vi "Utility Read From Register.vi"(7 "Unit Address (1)":u8=1, 8 "error in (no error)":errorcluster, 9 "Num Of Reg (1)":u16=1 min=1 step=1, 10 "Register Address (0)":u16, 11 "VISA resource name":refnum<visa-resource-name>) -> (0 "error out":errorcluster, 2 "Data":i16[](array[numeric]), 3 "VISA resource name out":refnum<visa-resource-name>)   [LabVIEW 2014, in "Eurotherm 35xx Series.lvlib"]
doc: "This VI reads value from specified registers of specified unit."
uses:
  <instrlib>/Eurotherm 35xx Series/Eurotherm 35xx Series.lvlib
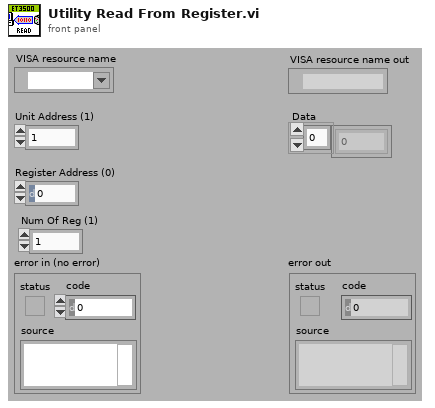
[diagram p1: front panel]
types:
  T1 = enum16{"By The Number of Bytes", "Copy Of the Sent Message"}
  T2 = cluster{"Read Buffer[0]":u8, "Read Buffer[1]":u8}
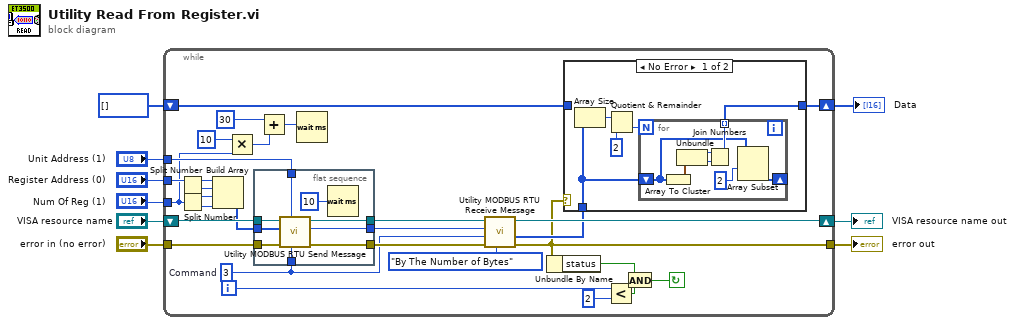
[diagram p0: block diagram]
diagram:
  n1 = while {
    tunnel: "Unit Address (1)" -> [w19]
    shift-right: [w35] -> w8
    shift-left: "VISA resource name" -> [w36]
    tunnel: "Register Address (0)" -> [w25]
    tunnel: "Num Of Reg (1)" -> [w10]
    shift-right: [w23] -> w6
    shift-left: u16[] [] -> [w22]
    tunnel: [w16] -> w2
    tunnel: "error in (no error)" -> [w15]
    i -> [w31]
    stop <- w33 continue-if-true
    w32 = u8 3  # Command
    n2 = Split Number(x=w25) -> (hi(x)=w27:u8, lo(x)=w26:u8)
    n3 = Split Number(x=w10) -> (hi(x)=w21:u8, lo(x)=w20:u8)
    n4 = Build Array(w27, w26, w21, w20) -> (w28:u8[])
    n5 = Multiply(x=u32 10, y=w10) -> (x*y=w13:u32)
    n6 = flat-sequence {
      tunnel: [w47] -> w38
      tunnel: [w46] -> w37
      tunnel: w36 -> [w45]
      tunnel: w32 -> [w44]
      tunnel: w28 -> [w43]
      tunnel: w19 -> [w42]
      tunnel: [w41] -> w17
      tunnel: w15 -> [w40]
      frame #0 {
        n7 = call <instrlib>:"Utility MODBUS RTU Send Message.vi"("Command (0)"=w44, "Unit Address (1)"=w42, "error in (no error)"=w40, "Message (empty array)"=w43, "VISA resource name"=w45) -> ("error out"=w47:errorcluster, "Length Of Sent MSG"=w41:u8, "VISA resource name out"=w46:refnum<visa-resource-name>)  [unwired: 4 in]
        n8 = Wait (ms)(milliseconds to wait=u32 10) -> ()  [unwired: 1 out]
      }
    }
    n9 = Add(x=u32 30 ("milliseconds to wait"), y=w13) -> (x+y=w12:u32)
    n10 = Wait (ms)(milliseconds to wait=w12) -> ()  [unwired: 1 out]
    n11 = call <instrlib>:"Utility MODBUS RTU Receive Message.vi"("Receive Message Type (0: By The Number Of Bytes)"=T1."By The Number of Bytes" ("Receive Message Type"), "error in (no error)"=w38, "Sent Command (0)"=w32, "Length Of Sent MSG (0)"=w17, "VISA resource name"=w37) -> ("error out"=w16:errorcluster, "Read Buffer"=w24:u8[], "VISA resource name out"=w35:refnum<visa-resource-name>)  [unwired: 4 in]
    n12 = Unbundle By Name(w16) -> ("status"=w34:bool)
    n13 = case shown="No Error" w16 {
      tunnel: w24 -> [w52 _]
      tunnel: [w51 w60] -> w23
      tunnel: w22 -> [_ w60]
      frame No Error {
        n14 = Array Size(array=w52) -> (size(s)=w50:i32)
        n15 = Quotient & Remainder(x=w50, y=2) -> (floor(x/y)=w48:i32)  [unwired: 1 out]
        n16 = for {
          N: w48 -> [_]
          shift-right: [w54] -> _
          shift-left: w52 -> [w55]
          tunnel: [w56] -> w51 mode=indexing
          n17 = Array To Cluster(array=w55) -> (cluster=w59:T2)
          n18 = Unbundle(w59) -> ("Read Buffer[0]"=w57:u8, "Read Buffer[1]"=w58:u8)
          n19 = Join Numbers(hi=w57, lo=w58) -> ((hi.lo)=w56:u16)
          n20 = Array Subset(array=w55, index=2) -> (w54:u8[])  [unwired: 1 in]
        }
      }
      frame Error {
      }
    }
    n21 = Less?(x=w31, y=2) -> (x < y?=w30:bool)
    n22 = And(x=w34, y=w30) -> (x .and. y?=w33:bool)
  }
  "error out" <- w2
  "VISA resource name out" <- w8
  "Data" <- w6
